vi "PathPlanner_Trajectory_GetNextRotationTargetIdx.vi"(9 "Starting Index":i32, 11 "PathPlannerPath":T1={"Reversed"=FALSE, "RotationTargets"=[], "ConstraintZones"=[], "EventMarkers"=[], "GlobalConstraints"={"MaxVelocityMps;"=0.0, "MaxAccelerationMpsSq;"=0.0, "MaxAngularVelRadPsEc;"=0.0, "MaxAngularAccRadPSecSq"=0.0, "Exists"=FALSE, "Unlimited"=FALSE, "NominalVoltageVolts"=12.0}, "GoalEndState"={"VelocityMPS"=0.0, "Rotation"={"VALUE"=0.0, "COS"=1.0, "SIN"=0.0}}, "AllPoints"=[], "Name"="", "Waypoints"=[], "PointTowardsZones"=[], "IdealStartingState"={"VelocityMPS"=0.0, "Rotation"={"VALUE"=1.0, "COS"=0.0, "SIN"=0.0}}, "IsChoreoPath"=FALSE, "PreventFlipping"=FALSE} {"IdealStartingState"."Rotation"."SIN" format="%13.4f"; "IdealStartingState"."Rotation"."COS" format="%13.4f"; "IdealStartingState"."Rotation"."VALUE" format="%13.4f"; "PointTowardsZones"."TargetPosition"."Y" format="%14.3f"; "PointTowardsZones"."TargetPosition"."X" format="%14.3f"; "PointTowardsZones"."RotationOffset"."SIN" format="%13.4f"; "PointTowardsZones"."RotationOffset"."COS" format="%13.4f"; "PointTowardsZones"."RotationOffset"."VALUE" format="%13.4f"; "Waypoints"."nextControl"."Y" format="%14.3f"; "Waypoints"."nextControl"."X" format="%14.3f"; "Waypoints"."anchor"."Y" format="%14.3f"; "Waypoints"."anchor"."X" format="%14.3f"; "Waypoints"."prevControl"."Y" format="%14.3f"; "Waypoints"."prevControl"."X" format="%14.3f"; "AllPoints"."RotationTarget"."rotation"."SIN" format="%13.4f"; "AllPoints"."RotationTarget"."rotation"."COS" format="%13.4f"; "AllPoints"."RotationTarget"."rotation"."VALUE" format="%13.4f"; "AllPoints"."Position"."Y" format="%14.3f"; "AllPoints"."Position"."X" format="%14.3f"; "GoalEndState"."Rotation"."SIN" format="%13.4f"; "GoalEndState"."Rotation"."COS" format="%13.4f"; "GoalEndState"."Rotation"."VALUE" format="%13.4f"; "RotationTargets"."rotation"."SIN" format="%13.4f"; "RotationTargets"."rotation"."COS" format="%13.4f"; "RotationTargets"."rotation"."VALUE" format="%13.4f"}) -> (1 "Found":bool, 3 "Idx":i32)   [LabVIEW 2019, in "PathPlanner24.lvlib"]
doc: "Inputs: \n - path - cluster - path definition\n\nOutputs:\n - NextRotationTargetIndex - integer - \n - Found - boolean - rotation was found"
uses:
  PathPlanner24.lvlib
  <vilib>/Rock Robotics/WPI/ThirdParty/JAS_Junk/TrajLib/TypeDef/TRANSLATION2D.ctl
  <vilib>/Rock Robotics/WPI/ThirdParty/JAS_Junk/TrajLib/Trajectory_Library.lvlib
  <vilib>/Rock Robotics/WPI/ThirdParty/JAS_Junk/TrajLib/TypeDef/ROTATION2D.ctl
  TypeDef/PathPlannerPathConstraints.ctl
  TypeDef/PathPlannerRotationTarget.ctl
  TypeDef/PathPlannerConstraintsZone.ctl
  TypeDef/PathPlannerCommandUtil.ctl
  TypeDef/PathPlannerEventMarker.ctl
  TypeDef/PathPlannerGoalEndState.ctl
  TypeDef/PathPlannerPathPoint.ctl
  TypeDef/PathPlannerPath.ctl
  ENum/PathPlanner_CommandUtilType_ENUM.ctl
  TypeDef/PathPlannerWaypoint.ctl
  TypeDef/PathPlannerPointTowardsZone.ctl
  TypeDef/PathPlannerIdealStartingState.ctl
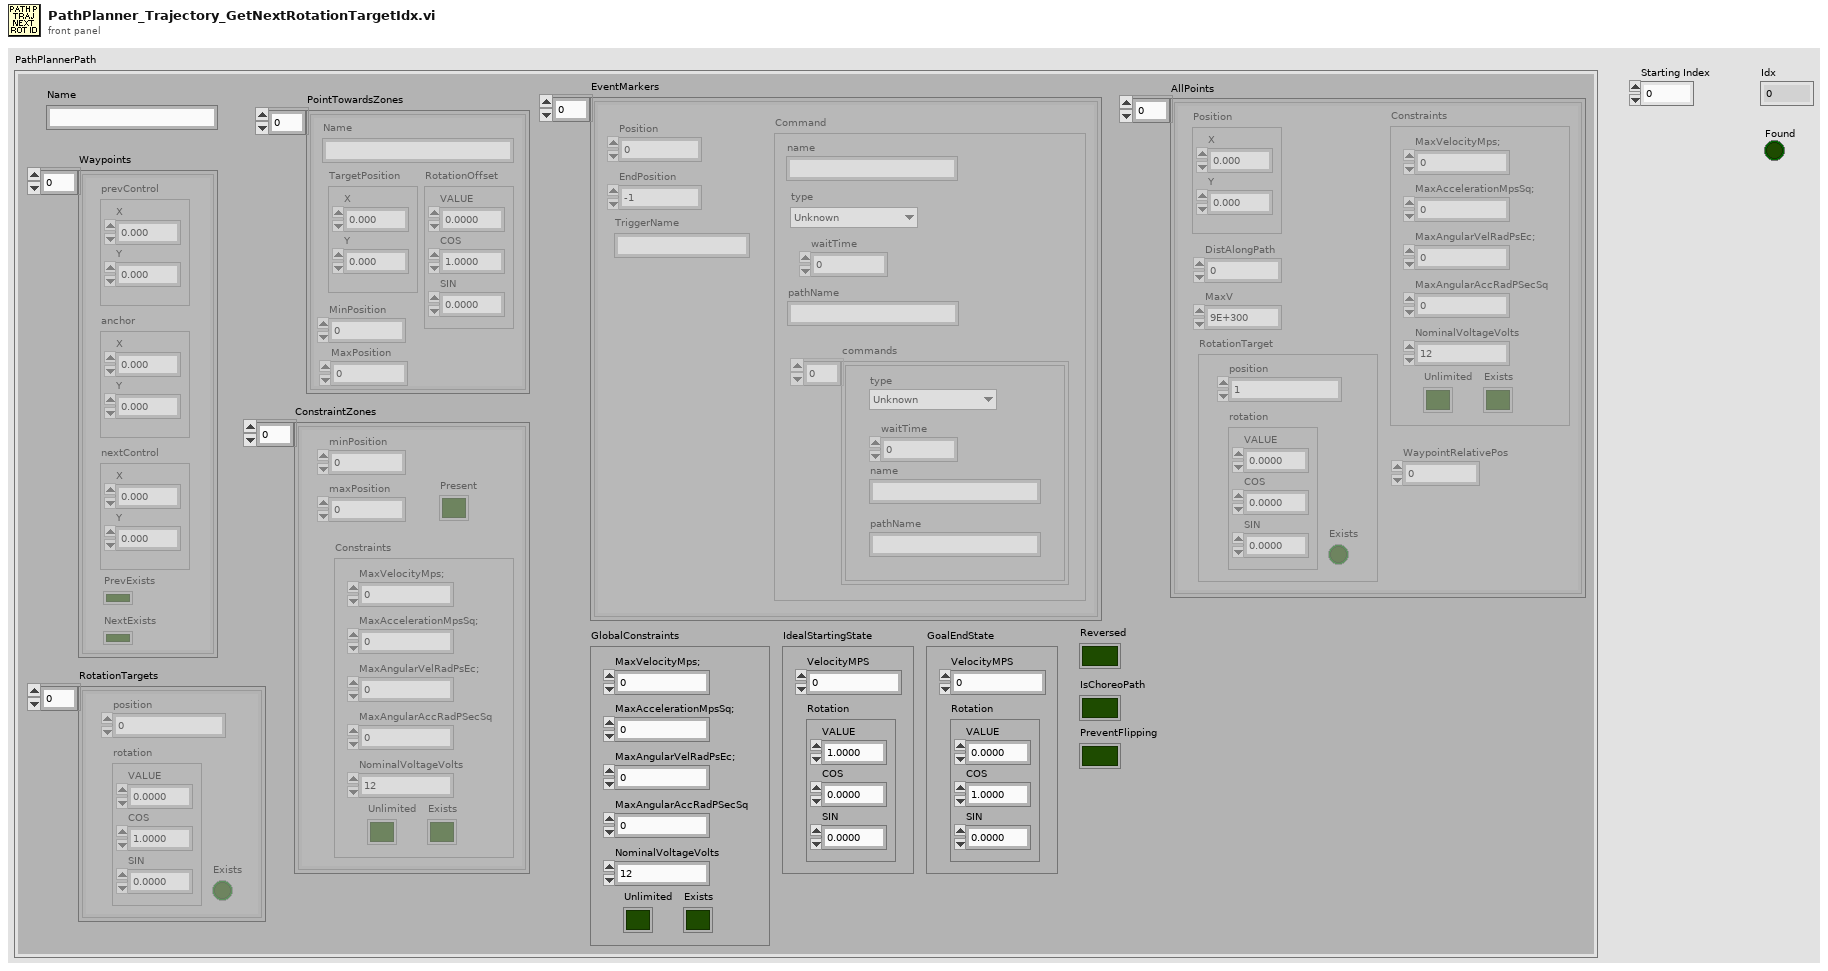
[diagram p1: front panel]
types:
  T1 = typedef "PathPlanner24.lvlib/PathPlannerPath.ctl" = cluster{"Reversed":bool, "RotationTargets":T2[], "ConstraintZones":T4[], "EventMarkers":T6[], "GlobalConstraints":T5, "GoalEndState":T9, "AllPoints":T10[], "Name":string, "Waypoints":T12[], "PointTowardsZones":T13[], "IdealStartingState":T14, "IsChoreoPath":bool, "PreventFlipping":bool}
  T2 = typedef "PathPlanner24.lvlib/PathPlannerRotationTarget.ctl" = cluster{"position":dbl, "rotation":T3, "Exists":bool}
  T3 = typedef "Trajectory_Library.lvlib/ROTATION2D.ctl" = cluster{"VALUE":dbl, "COS":dbl, "SIN":dbl}
  T4 = typedef "PathPlanner24.lvlib/PathPlannerConstraintsZone.ctl" = cluster{"minPosition":dbl, "maxPosition":dbl, "Constraints":T5, "Present":bool}
  T5 = typedef "PathPlanner24.lvlib/PathPlannerPathConstraints.ctl" = cluster{"MaxVelocityMps;":dbl, "MaxAccelerationMpsSq;":dbl, "MaxAngularVelRadPsEc;":dbl, "MaxAngularAccRadPSecSq":dbl, "Exists":bool, "Unlimited":bool, "NominalVoltageVolts":dbl}
  T6 = typedef "PathPlanner24.lvlib/PathPlannerEventMarker.ctl" = cluster{"Position":dbl, "Command":T7, "TriggerName":string, "EndPosition":dbl}
  T7 = typedef "PathPlanner24.lvlib/PathPlannerCommandUtil.ctl" = cluster{"waitTime":dbl, "name":string, "pathName":string, "commands":cluster{"type":T8, "waitTime":dbl, "name":string, "pathName":string}[], "type":T8}
  T8 = typedef "PathPlanner24.lvlib/PathPlanner_CommandUtilType_ENUM.ctl" = enum16{"Unknown", "Wait", "Named", "Path", "Sequential", "Parallel", "Race", "Deadline"}
  T9 = typedef "PathPlanner24.lvlib/PathPlannerGoalEndState.ctl" = cluster{"VelocityMPS":dbl, "Rotation":T3}
  T10 = typedef "PathPlanner24.lvlib/PathPlannerPathPoint.ctl" = cluster{"Position":T11, "DistAlongPath":dbl, "MaxV":dbl, "Constraints":T5, "RotationTarget":T2, "WaypointRelativePos":dbl}
  T11 = typedef "Trajectory_Library.lvlib/TRANSLATION2D.ctl" = cluster{"X":dbl, "Y":dbl}
  T12 = typedef "PathPlanner24.lvlib/PathPlannerWaypoint.ctl" = cluster{"prevControl":T11, "anchor":T11, "nextControl":T11, "PrevExists":bool, "NextExists":bool}
  T13 = typedef "PathPlanner24.lvlib/PathPlannerPointTowardsZone.ctl" = cluster{"RotationOffset":T3, "Name":string, "TargetPosition":T11, "MinPosition":dbl, "MaxPosition":dbl}
  T14 = typedef "PathPlanner24.lvlib/PathPlannerIdealStartingState.ctl" = cluster{"VelocityMPS":dbl, "Rotation":T3}
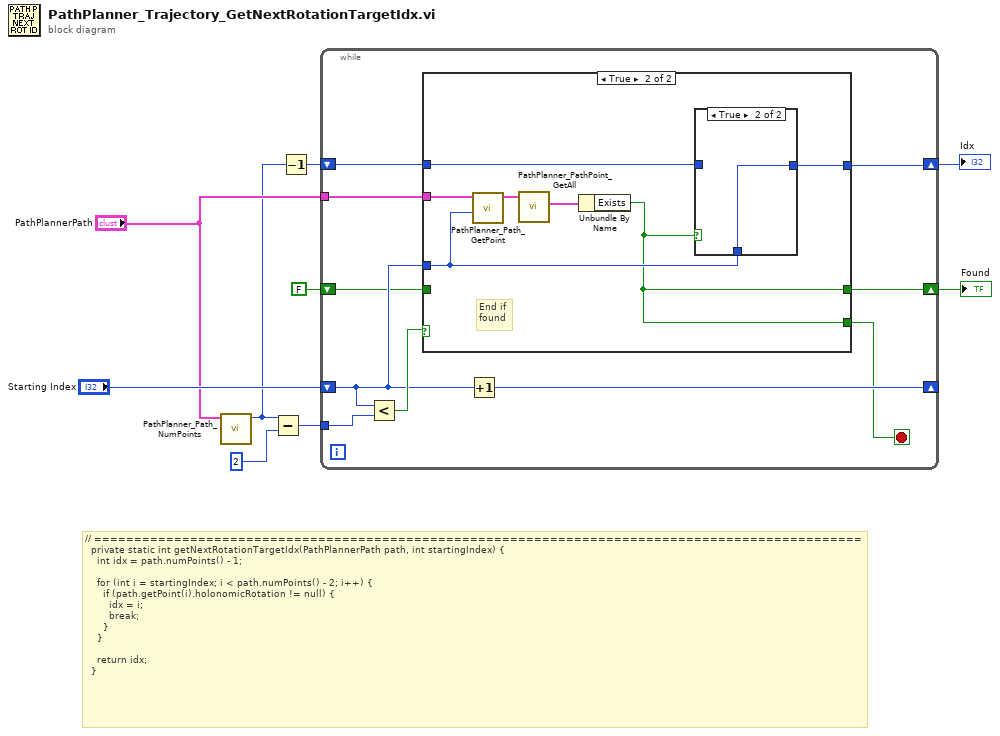
[diagram p0: block diagram]
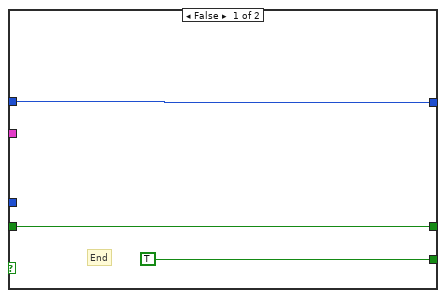
[diagram p2: hidden frame]
diagram:
  # "// ================================================================================================\n  private static int getNextRotationTargetIdx(PathPlannerPath path, int startingIndex) {\n    int idx = path.numPoints() - 1;\n\n    for (int i = startingIndex; i < path.numPoints() - 2; i++) {\n      if (path.getPoint(i).holonomicRotation != null) {\n        idx = i;\n        break;\n      }\n    }\n\n    return idx;\n  }"
  n1 = call "PathPlanner_Path_NumPoints.vi"("PathPlannerPath"="PathPlannerPath") -> ("NumPoints"=w1:i32)  [unwired: 10 in]
  n2 = Subtract(x=w1, y=2) -> (x-y=w8:i32)
  n3 = Decrement(x=w1) -> (x-1=w2:i32)
  n4 = while {
    tunnel: "PathPlannerPath" -> [w19]
    shift-right: [w16] -> _
    shift-left: "Starting Index" -> [w11]
    tunnel: w8 -> [w15]
    shift-right: [w18] -> w6
    shift-left: w2 -> [w17]
    shift-right: [w12] -> w4
    shift-left: FALSE ("HolonomicRotationExists") -> [w10]
    stop <- w13 stop-if-true
    n5 = Less?(x=w11, y=w15) -> (x < y?=w14:bool)
    n6 = case shown="True" w14 {
      tunnel: w19 -> [_ w29]
      tunnel: w11 -> [_ w27]
      tunnel: [w22 w26] -> w18
      tunnel: [w20 w23] -> w12
      tunnel: w17 -> [w22 w25]
      tunnel: [TRUE ("HolonomicRotationExists") w23] -> w13
      tunnel: w10 -> [w20 _]
      frame False {
        # "End"
      }
      frame True {
        # "End if\nfound"
        n7 = call "PathPlanner_Path_GetPoint.vi"("Index"=w27, "PathPlannerPath"=w29) -> ("Point"=w28:T10)  [unwired: 9 in]
        n8 = call "PathPlanner_PathPoint_GetAll.vi"("PathPlannerPoint"=w28) -> ("RotationTarget"=w24:T2)  [unwired: 5 in, 5 out]
        n9 = Unbundle By Name(w24) -> ("Exists"=w23:bool)
        n10 = case shown="True" w23 {
          tunnel: w27 -> [_ w31]
          tunnel: [w30 w31] -> w26
          tunnel: w25 -> [w30 _]
          frame False {
          }
          frame True {
          }
        }
      }
    }
    n11 = Increment(x=w11) -> (x+1=w16:i32)
  }
  "Idx" <- w6
  "Found" <- w4
